vi "check_pass_range.vi"(9 "Output V avg range":dbl, 10 "Output V avg center point":dbl, 11 "Output V avg":dbl) -> (3 "Pass range?":bool)   [LabVIEW 2019]
doc: "Checks if the Output V avg input falls within the range of Output V avg center point +- Output V avg range"
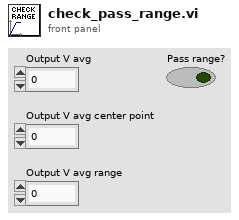
[diagram p1: front panel]
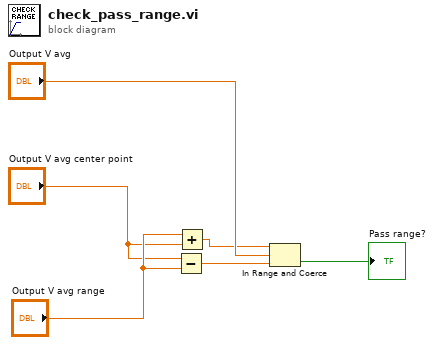
[diagram p0: block diagram]
diagram:
  n1 = Subtract(x="Output V avg center point", y="Output V avg range") -> (x-y=w1:dbl)
  n2 = Add(x="Output V avg range", y="Output V avg center point") -> (x+y=w4:dbl)
  n3 = In Range and Coerce(upper limit=w4, x="Output V avg", lower limit=w1) -> (In Range?=→"Pass range?":bool)  [unwired: 1 out]
